vi "In_S1F11.vi"(8 "error in (no error)":errorcluster, 11 "S1 Message Class in":refnum<class "S1 Message Class.lvclass">) -> (0 "error out":errorcluster, 1 "OK?":bool, 2 "Status Variable ID(SVID)":u32[](array[numeric]), 3 "S1 Message Class out":refnum<class "S1 Message Class.lvclass">)   [LabVIEW 2020, in "SECS Communication.lvlib" / "S1 Message Class.lvclass"]
uses:
  S1 Message Class.lvclass
  D:/Dropbox/SECS/SECS_GEM v1.0.6/Com/SECS Communication/SECS-II Class/SECS-II Class.lvclass
  SECS-II Class/SECS-II Class.lvclass/SECS-II Class.ctl
  SECS-II Class/Variant To Data_U4.vi
  SECS-II Class/SECS-II Class.lvclass
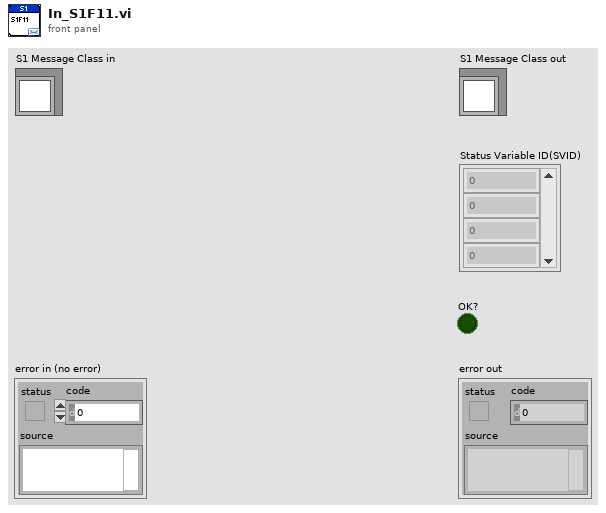
[diagram p1: front panel]
types:
  T1 = typedef "SECS Communication.lvlib/SECS-II Class.lvclass/Message Data.ctl" = cluster{"Index":i32, "Data Item Format":T2, "Format Code":T3, "Parent Index":i32, "Child Index":i32[], "Data":variant}
  T2 = typedef "SECS Communication.lvlib/SECS-II Class.lvclass/Data Item Format.ctl" = enum16{"Data Type", "Value"}
  T3 = typedef "SECS Communication.lvlib/SECS-II Class.lvclass/Format Code.ctl" = enum16{"L", "A", "B", "Boolean", "J", "I1", "I2", "I4", "I8", "U1", "U2", "U4", "U8", "F4", "F8", "Char"}
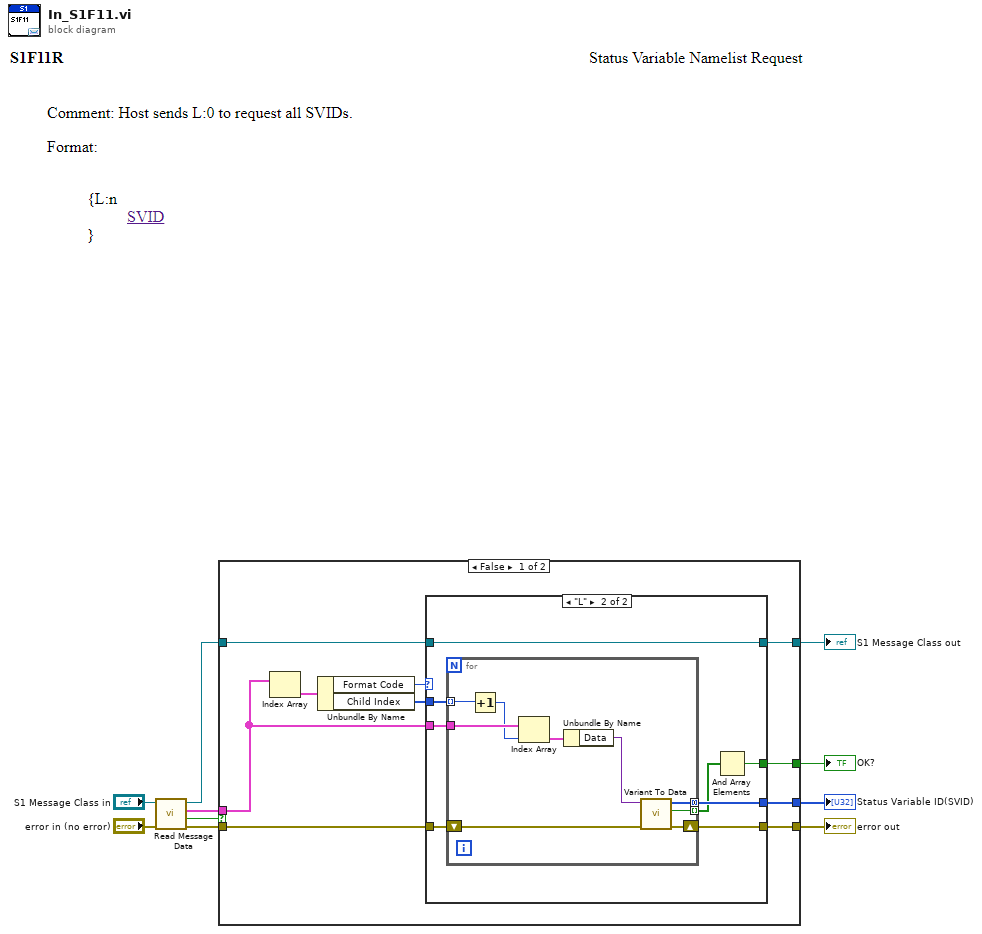
[diagram p0: block diagram]
diagram:
  n1 = call "Read Message Data.vi"("error in (no error)"="error in (no error)", "SECS-II Class in"="S1 Message Class in") -> ("error out"=w9:errorcluster, "Empty?"=w1:bool, "Message Data"=w10:T1[], "SECS-II Class out"=w8:refnum<class "S1 Message Class.lvclass">)  [unwired: 6 in]
  n2 = case shown="False" w1 {
    tunnel: w10 -> [w18 _]
    tunnel: w9 -> [w17 w40]
    tunnel: w8 -> [w15 w41]
    tunnel: [w14 w40] -> w5
    tunnel: [w13 _] -> w4
    tunnel: [w12 w41] -> w3
    tunnel: [w11 _] -> w2
    frame False {
      n3 = Index Array(array=w18) -> (element=w20:T1)  [unwired: 1 in]
      n4 = Unbundle By Name(w20) -> ("Format Code"=w16:T3, "Child Index"=w19:i32[])
      n5 = case shown="\"L\"" w16 {
        tunnel: w19 -> [_ w30]
        tunnel: w18 -> [_ w29]
        tunnel: w17 -> [w21 w28]
        tunnel: [w21 w27] -> w14
        tunnel: [_ w26] -> w13
        tunnel: w15 -> [w22 w25]
        tunnel: [w22 w25] -> w12
        tunnel: [_ w23] -> w11
        frame Default {
        }
        frame "L" {
          n6 = for {
            tunnel: w30 -> [w38] mode=indexing
            tunnel: w29 -> [w39]
            shift-right: [w32] -> w27
            shift-left: w28 -> [w35]
            tunnel: [w33] -> w26 mode=concatenating
            tunnel: [w31] -> w24 mode=indexing
            n7 = Increment(x=w38) -> (x+1=w37:i32)
            n8 = Index Array(array=w39, index=w37) -> (element=w36:T1)
            n9 = Unbundle By Name(w36) -> ("Data"=w34:variant)
            n10 = call-poly "Variant To Data.vi"("error in (no error)"=w35, "Variant"=w34) -> ("error out"=w32:errorcluster, "OK?"=w31:bool, "Data"=w33:u32[])  [unwired: 7 in]
          }
          n11 = And Array Elements(Boolean array=w24) -> (logical AND=w23:bool)
        }
      }
    }
    frame True {
    }
  }
  "error out" <- w5
  "S1 Message Class out" <- w3
  "Status Variable ID(SVID)" <- w4
  "OK?" <- w2
